vi "algorithm52.vi"(10 "String":string) -> (2 "y":i32)   [LabVIEW 2017]
panel:
  out "Array":i32[][](array[numeric])
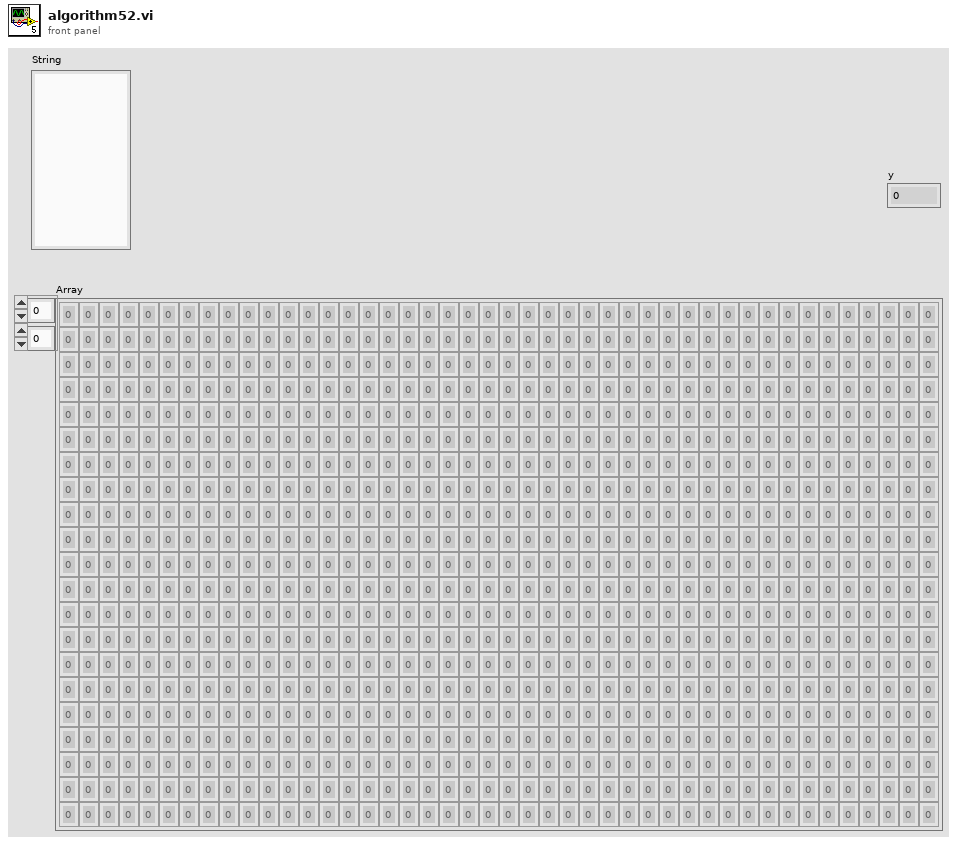
[diagram p1: front panel]
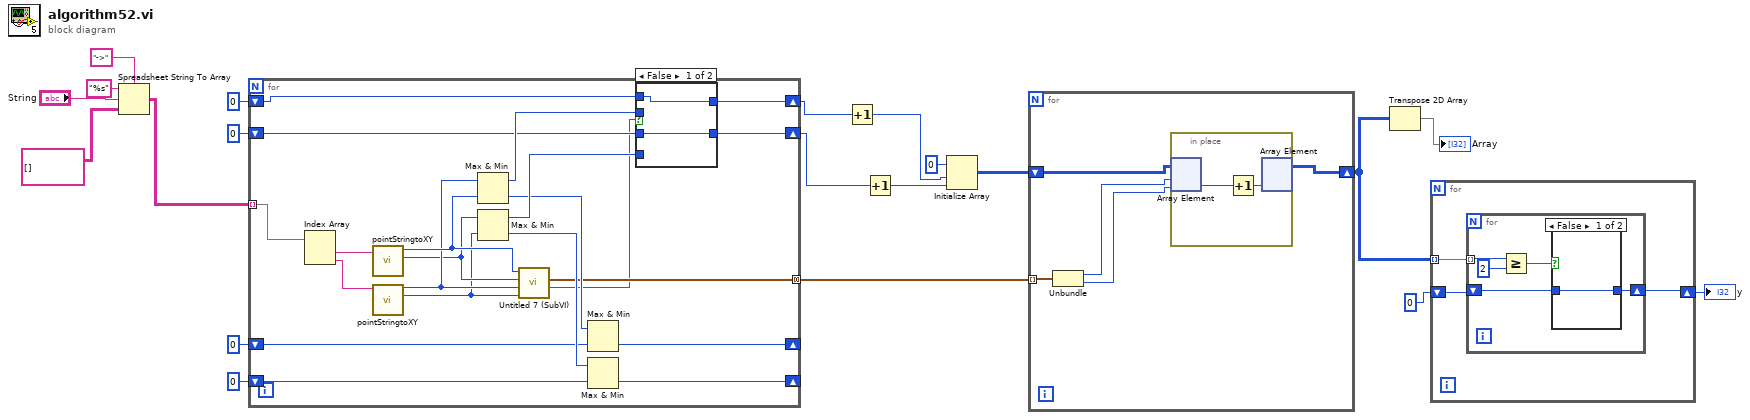
[diagram p0: block diagram]
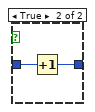
[diagram p2: hidden frame]
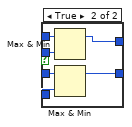
[diagram p3: hidden frame]
diagram:
  n1 = Spreadsheet String To Array(delimiter (Tab)="->", format string="%s", spreadsheet string="String", array type (2D Dbl)=string[][] []) -> (array=w16:string[][])
  n2 = for {
    tunnel: w16 -> [w41] mode=indexing
    shift-right: [w30] -> _
    shift-left: 0 -> [w29]
    shift-right: [w28] -> _
    shift-left: 0 -> [w27]
    shift-right: [w26] -> w12
    shift-left: 0 -> [w25]
    shift-right: [w24] -> w11
    shift-left: 0 -> [w23]
    tunnel: [w22] -> w10 mode=concatenating
    n3 = Index Array(array=w41) -> (element #1=w40:string, element #2=w39:string)  [unwired: 2 in]
    n4 = call "pointStringtoXY.vi"("stringPoint"=w40) -> ("y"=w36:i32, "x"=w38:i32)  [unwired: 9 in]
    n5 = call "pointStringtoXY.vi"("stringPoint"=w39) -> ("y"=w35:i32, "x"=w37:i32)  [unwired: 9 in]
    n6 = Max & Min(x=w37, y=w38) -> (max(x,y)=w34:i32, min(x,y)=w32:i32)
    n7 = Max & Min(x=w36, y=w35) -> (max(x,y)=w33:i32, min(x,y)=w31:i32)
    n8 = call "Untitled 7 (SubVI).vi"("y 2"=w35, "x 2"=w37, "y 1"=w36, "x 1"=w38) -> ("Boolean"=w21:bool, "Array"=w22:cluster{"x 1":i32, i32}[])  [unwired: 6 in]
    n9 = Max & Min(x=w32, y=w29) -> (min(x,y)=w30:i32)  [unwired: 1 out]
    n10 = Max & Min(x=w31, y=w27) -> (min(x,y)=w28:i32)  [unwired: 1 out]
    n11 = case shown="False" w21 {
      tunnel: w34 -> [_ w49]
      tunnel: w33 -> [_ w48]
      tunnel: [w43 w47] -> w26
      tunnel: w25 -> [w43 w46]
      tunnel: [w42 w45] -> w24
      tunnel: w23 -> [w42 w44]
      frame False {
      }
      frame True {
        n12 = Max & Min(x=w46, y=w49) -> (max(x,y)=w47:i32)  [unwired: 1 out]
        n13 = Max & Min(x=w44, y=w48) -> (max(x,y)=w45:i32)  [unwired: 1 out]
      }
    }
  }
  n14 = Increment(x=w12) -> (x+1=w6:i32)
  n15 = Increment(x=w11) -> (x+1=w5:i32)
  n16 = Initialize Array(0 ("element"), w6, w5) -> (w9:i32[][])
  n17 = for {
    tunnel: w10 -> [w54] mode=indexing
    shift-right: [w50] -> w2
    shift-left: w9 -> [w53]
    n18 = Unbundle(w54) -> ("x 1"=w52:i32, w51:i32)
    n19 = in-place {
      n20 = in-place-array #1(w53, w52, w51) -> (w56:i32)
      n21 = Increment(x=w56) -> (x+1=w55:i32)
      n22 = in-place-array #1(w55) -> (w50:i32[][])  [unwired: 2 out]
    }
  }
  n23 = Transpose 2D Array(2D array=w2) -> (transposed array=→"Array":i32[][])
  n24 = for {
    tunnel: w2 -> [w59] mode=indexing
    shift-right: [w58] -> w7
    shift-left: 0 ("y") -> [w57]
    n25 = for {
      tunnel: w59 -> [w64] mode=indexing
      shift-right: [w61] -> w58
      shift-left: w57 -> [w60]
      n26 = Greater Or Equal?(x=w64, y=2) -> (x >= y?=w62:bool)
      n27 = case shown="False" w62 {
        tunnel: [w65 w67] -> w61
        tunnel: w60 -> [w65 w66]
        frame False {
        }
        frame True {
          n28 = Increment(x=w66) -> (x+1=w67:i32)
        }
      }
    }
  }
  "y" <- w7
